vi "Main.vi"(11 "Module Admin":refnum<class "Delacor_lib_QMH_Module Admin.lvclass">) -> ()   [LabVIEW 2025, in "ATM Module.lvlib"]
doc: "ATM machine made with a DQMH module.\n\nTakes user input in the form of a PIN to verify account.\n\nShows balance. Facilitates withdraw, deposit, and \"Fast Cash\" $50 withdrawals."
uses:
  ATM Module.lvlib
  <vilib>/Delacor/Delacor QMH/Libraries/Module Admin_class/Delacor_lib_QMH_Module Admin.lvclass
  Controls/FP Data Refs.ctl
  Module Data--cluster.ctl
  Stop Argument--cluster.ctl
  <vilib>/Delacor/Delacor QMH/Libraries/Message Queue_class/Delacor_lib_QMH_Message Queue.lvclass/Delacor_lib_QMH_Message Queue.ctl
  <vilib>/Delacor/Delacor QMH/Libraries/Module Admin_class/Delacor_lib_QMH_Module Admin.lvclass/Delacor_lib_QMH_Module Admin.ctl
  <vilib>/Utility/miscctls.llb/LVPointTypeDef.ctl
  <vilib>/Delacor/Delacor QMH/Libraries/Message Queue_class/Delacor_lib_QMH_Enqueue Message (Single).vi
  <vilib>/Delacor/Delacor QMH/Libraries/Module Admin_class/Delacor_lib_QMH_Get External Launch.vi
  <vilib>/Delacor/Delacor QMH/Libraries/Message Queue_class/Delacor_lib_QMH_Message Queue.lvclass
panel:
  in  "Enter":bool
  in  "User Input":string
  in  "Right Buttons":T1
  out "Right Menu":T2
  in  "Left Buttons":T1
  out "Left Menu":T2
  in  "Card Simulator":bool
  out "ATM Messages":string
  out "error out":errorcluster
  out "Status":string
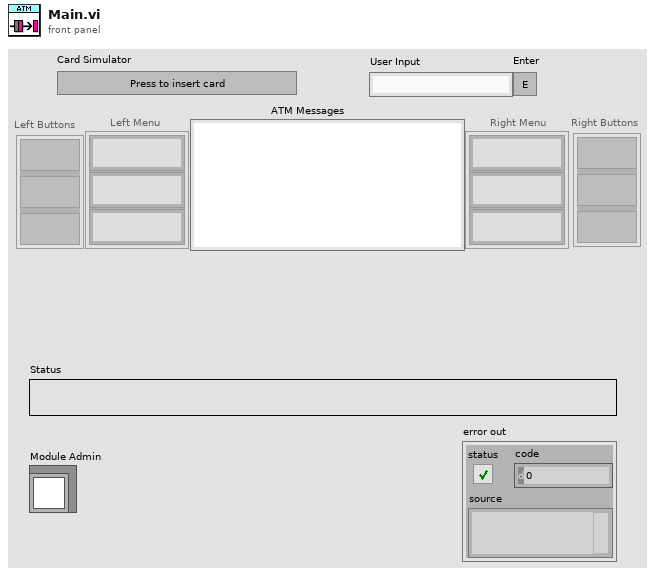
[diagram p1: front panel]
types:
  T1 = cluster{"Func Button":bool, "Func Button 2":bool, "Func Button 3":bool}
  T2 = cluster{"RFS String":string, "RFS String 2":string, "RFS String 3":string}
  T3 = typedef "FP Data Refs.ctl" = cluster{"User Input":refnum<vi>, "Right Buttons":refnum<vi>, "Right Menu":refnum<vi>, "Left Buttons":refnum<vi>, "Left Menu":refnum<vi>, "Enter":refnum<vi>}
  T4 = typedef "ATM Module.lvlib/Request Events--cluster.ctl" = cluster{"Stop Module":refnum<user-event>, "Show Panel":refnum<user-event>, "Hide Panel":refnum<user-event>, "Get Module Execution Status":refnum<user-event>, "Show Diagram":refnum<user-event>, "Private.Reset Timer":refnum<user-event>}
  T5 = typedef "ATM Module.lvlib/Module Data--cluster.ctl" = cluster{"Status":string, "Account PIN":string}
  T6 = enum32{"invalid lock state", "Not Locked", "Locked (No Password)", "Password-protected"}
  T7 = typedef "ATM Module.lvlib/Stop Argument--cluster.ctl" = cluster{"Origin":string, "Exit via Stop Module Req?":bool, "Wait for Module to stop?":bool}
  T8 = typedef "LVPointTypeDef.ctl" = cluster{"Horizontal":i16, "Vertical":i16}
  T9 = enum32{"Invalid", "Standard", "Closed", "Hidden", "Minimized", "Maximized"}
  T10 = enum8{"Enabled", "Disabled", "Disabled and Grayed Out"}
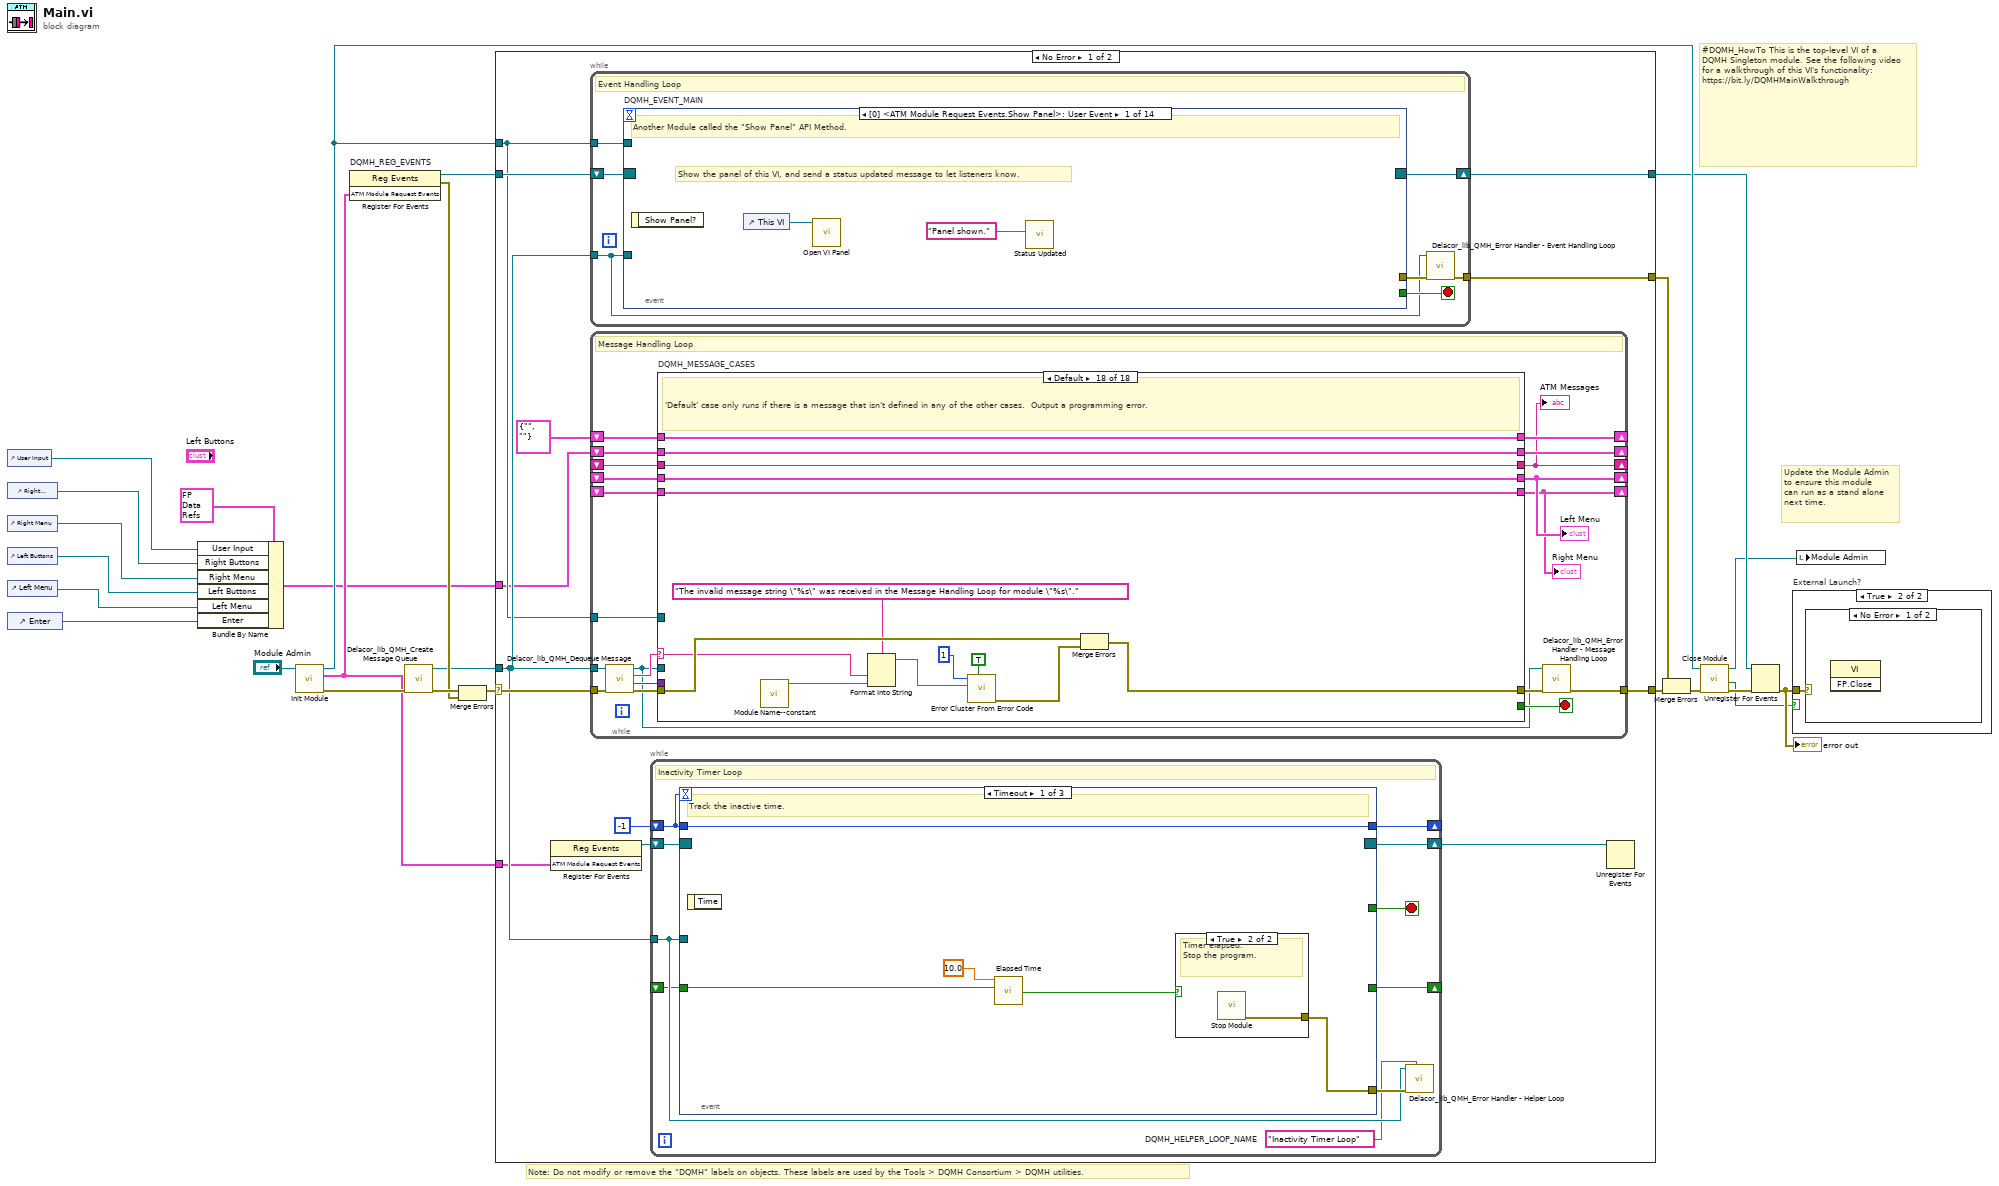
[diagram p0: block diagram]
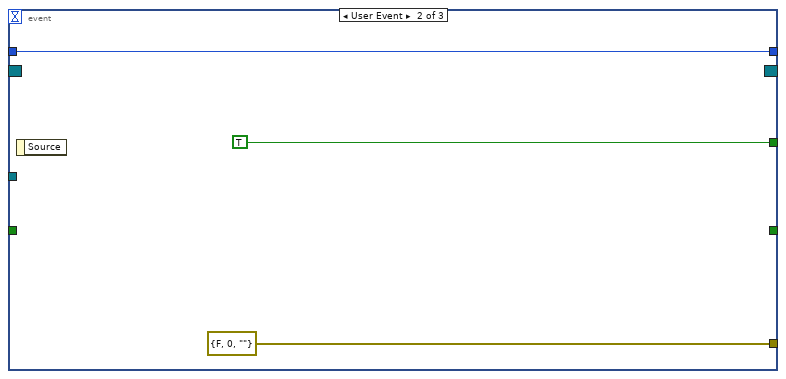
[diagram p3: hidden frame]
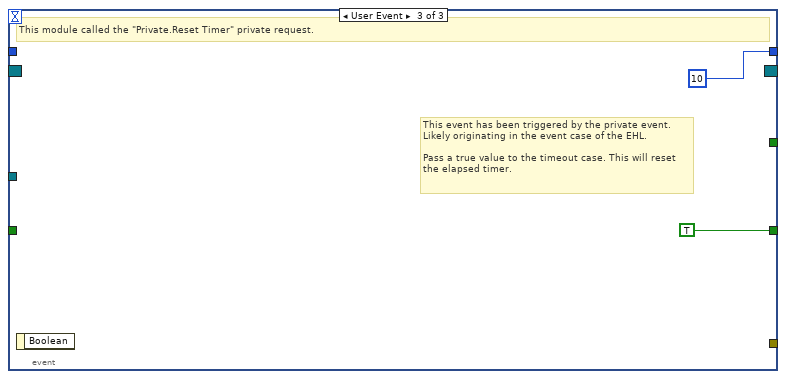
[diagram p4: hidden frame]
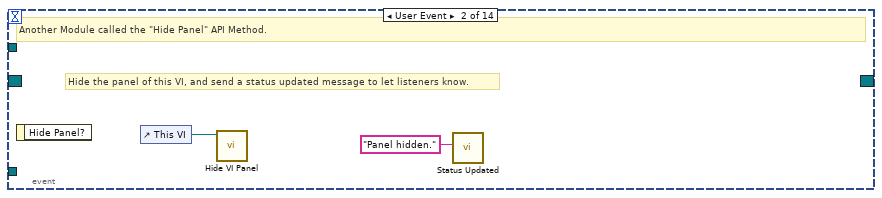
[diagram p5: hidden frame]
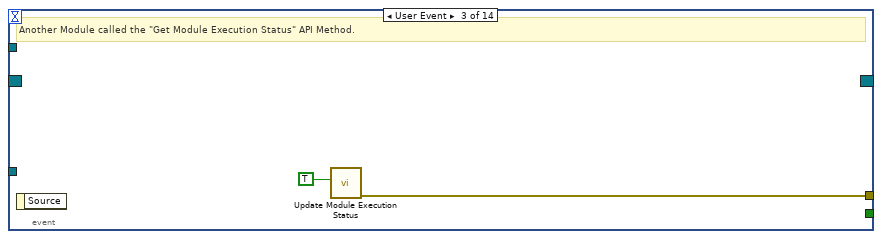
[diagram p6: hidden frame]
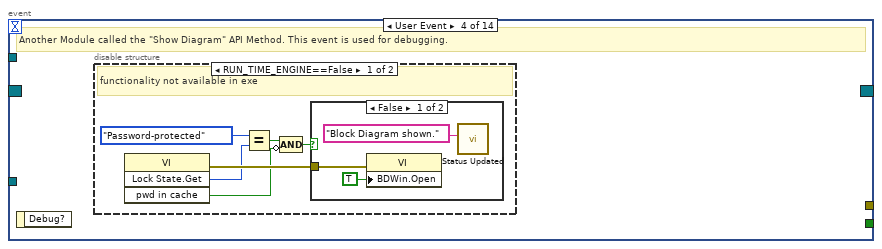
[diagram p7: hidden frame]
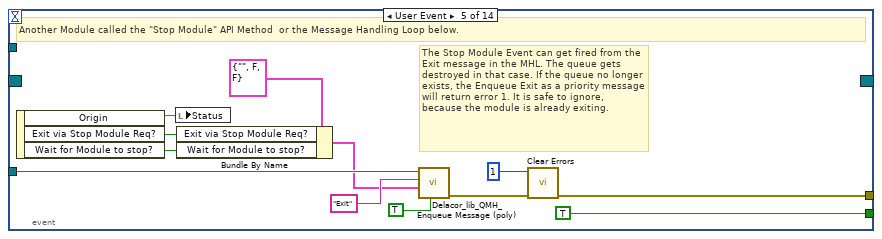
[diagram p10: hidden frame]
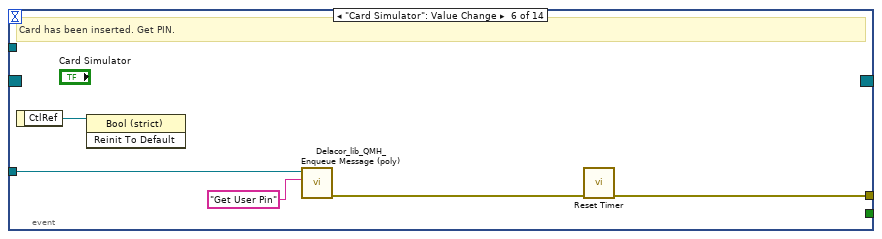
[diagram p11: hidden frame]
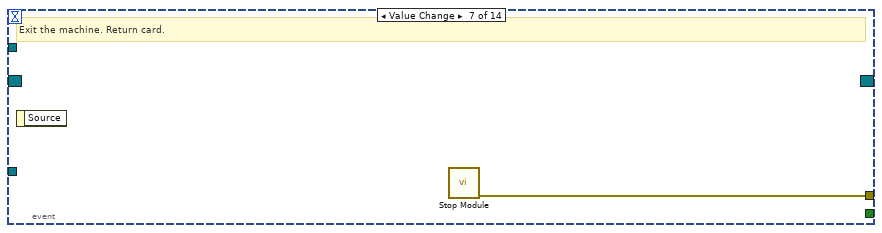
[diagram p12: hidden frame]
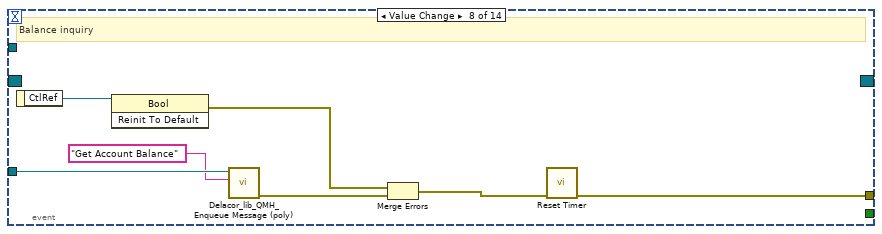
[diagram p13: hidden frame]
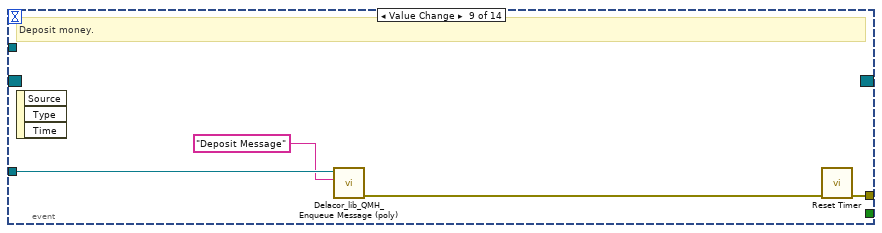
[diagram p14: hidden frame]
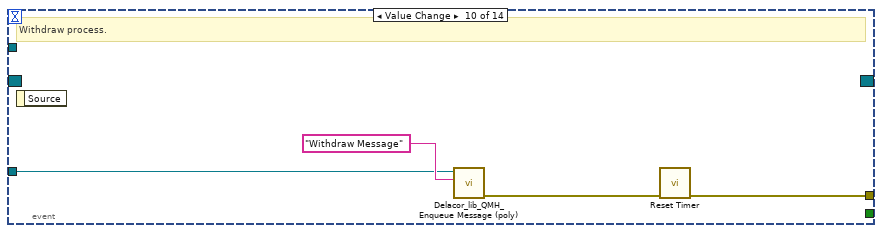
[diagram p15: hidden frame]
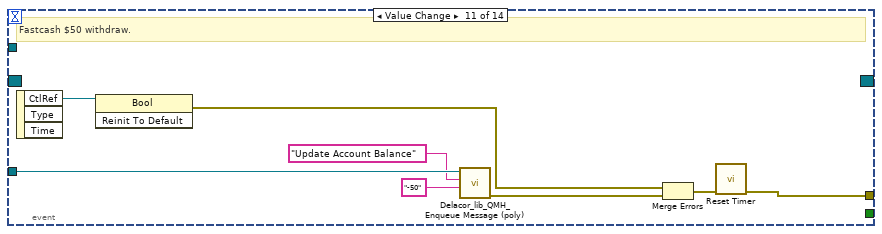
[diagram p16: hidden frame]
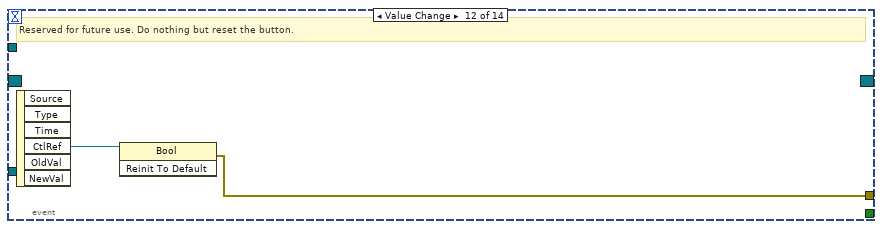
[diagram p17: hidden frame]
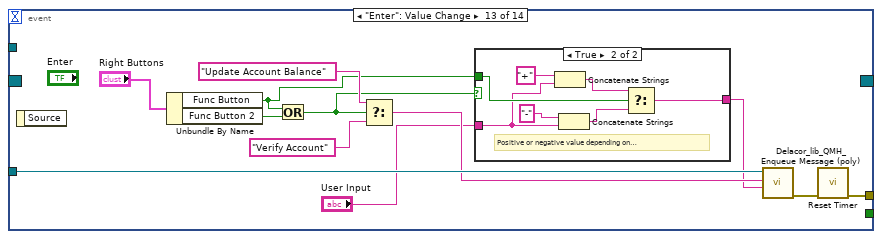
[diagram p18: hidden frame]
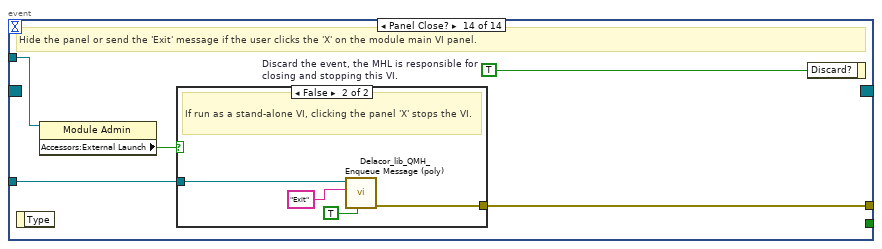
[diagram p20: hidden frame]
diagram:
  # "#DQMH_HowTo This is the top-level VI of a DQMH Singleton module. See the following video for a walkthrough of this VI's functionality: https://bit.ly/DQMHMainWalkthrough"
  # "Note: Do not modify or remove the \"DQMH\" labels on objects. These labels are used by the Tools > DQMH Consortium > DQMH utilities."
  # "Update the Module Admin to ensure this module can run as a stand alone next time."
  n1 = control-ref of="User Input"() -> (w8:refnum<vi>)
  n2 = control-ref of="Right Buttons"() -> (w7:refnum<vi>)
  n3 = control-ref of="Right Menu"() -> (w6:refnum<vi>)
  n4 = control-ref of="Left Buttons"() -> (w5:refnum<vi>)
  n5 = control-ref of="Left Menu"() -> (w4:refnum<vi>)
  n6 = control-ref of="Enter"() -> (w2:refnum<vi>)
  n7 = Bundle By Name(cluster=T3 {"User Input"=refnum, "Right Buttons"=refnum, "Right Menu"=refnum, "Left Buttons"=refnum, "Left Menu"=refnum, "Enter"=refnum}, "User Input"=w8, "Right Buttons"=w7, "Right Menu"=w6, "Left Buttons"=w5, "Left Menu"=w4, "Enter"=w2) -> (w3:T3)
  n8 = call "Init Module.vi"("Singleton Module Admin in"="Module Admin") -> ("error out"=w24:errorcluster, "ATM Module Request Events"=w9:T4, "Singleton Module Admin out"=w16:refnum<class "Delacor_lib_QMH_Module Admin.lvclass">)  [unwired: 8 in]
  n9 = register-events "DQMH_REG_EVENTS"(w9) -> (reference out=w14:refnum<event-registration>, error out=w17:errorcluster)  [unwired: 2 in]
  n10 = call <vilib>:"Delacor_lib_QMH_Create Message Queue.vi"("error in"=w24) -> ("error out"=w19:errorcluster, "Message Queue"=w13:refnum<class "Delacor_lib_QMH_Message Queue.lvclass">)  [unwired: 9 in]
  n11 = Merge Errors(w19, w17) -> (w18:errorcluster)
  n12 = case shown="No Error" w18 {
    selector: w18 -> [w36 w455]
    tunnel: [w38 w454] -> w25
    tunnel: [w35 w453] -> w15
    tunnel: w14 -> [w34 w453]
    tunnel: w13 -> [w33 w448]
    tunnel: [w37 _] -> w22
    tunnel: w16 -> [w32 w449]
    tunnel: w9 -> [w31 _]
    tunnel: w3 -> [w26 _]
    frame No Error {
      n13 = register-events ("DQMH_HELPER_REGFOREVENTS")(w31) -> (reference out=w29:refnum<event-registration>)  [unwired: 2 in, 1 out]
      n14 = while {
        tunnel: w33 -> [w60]
        shift-right: [w63] -> w35
        shift-left: w34 -> [w64]
        tunnel: [w65] -> w37
        tunnel: w32 -> [w61]
        stop <- w62 stop-if-true
        # "Event Handling Loop"
        n15 = event "DQMH_EVENT_MAIN" shown="[0] <ATM Module Request Events.Show Panel>: User Event" {
          selector: w64 -> [_ _ _ _ _ _ _ _ _ _ _ _ _ _]
          dyn-events: [_ _ _ _ _ _ _ _ _ _ _ _ _ _] -> w63
          timeout: _ -> [_ _ _ _ _ _ _ _ _ _ _ _ _ _]
          tunnel: [_ _ _ _ TRUE ("Discard?") _ _ _ _ _ _ _ _ _] -> w62
          tunnel: w60 -> [_ _ _ _ w89 w98 _ w105 w110 w112 w121 _ w132 w147]
          tunnel: [_ _ w72 _ w92 w94 w99 w102 w107 w111 w115 w123 w129 w149] -> w66
          tunnel: w61 -> [_ _ _ _ _ _ _ _ _ _ _ _ _ w146]
          event User Event {
            # "Show the panel of this VI, and send a status updated message to let listeners know."
            # "Another Module called the \"Show Panel\" API Method."
            n16 = event-data() -> ()  [unwired: 1 in, 1 out]
            n17 = control-ref of="This VI"() -> (w68:refnum<vi>)
            n18 = call "Open VI Panel.vi"("VI"=w68) -> ()  [unwired: 10 in, 1 out]
            n19 = call "Status Updated.vi"("Status"="Panel shown." ("format string")) -> ()  [unwired: 10 in, 1 out]
          }
          event User Event {
            # "Hide the panel of this VI, and send a status updated message to let listeners know."
            # "Another Module called the \"Hide Panel\" API Method."
            n20 = event-data() -> ()  [unwired: 1 in, 1 out]
            n21 = control-ref of="This VI"() -> (w70:refnum<vi>)
            n22 = call "Hide VI Panel.vi"("VI"=w70) -> ()  [unwired: 10 in, 1 out]
            n23 = call "Status Updated.vi"("Status"="Panel hidden." ("format string")) -> ()  [unwired: 10 in, 1 out]
          }
          event User Event {
            # "Another Module called the \"Get Module Execution Status\" API Method."
            n24 = event-data() -> ()  [unwired: 1 in, 1 out]
            n25 = call "Update Module Execution Status.vi"("Running?"=TRUE) -> ("error out"=w72:errorcluster)  [unwired: 10 in]
          }
          event User Event {
            # "Another Module called the \"Show Diagram\" API Method. This event is used for debugging."
            n26 = event-data() -> ()  [unwired: 1 in, 1 out]
            n27 = disable-structure shown="RUN_TIME_ENGINE==False" {
              frame condition #0 (active) {
                # "functionality not available in exe"
                n28 = invoke on="Invoke Node" class="VI" method="Lock State.Get"() -> (error out=w78:errorcluster, "Get Lock State"=w77:T6, "pwd in cache"=w74:bool)  [unwired: 4 in, 1 out]
                n29 = Equal?(x=T6."Password-protected", y=w77) -> (x = y?=w75:bool)
                n30 = Compound Arithmetic op=AND(w75, invert w74) -> (w73:bool)
                n31 = case shown="False" w73 {
                  tunnel: w78 -> [w81 _]
                  frame False {
                    n32 = property on="Property Node" class="VI"(error in=w81, "BDWin.Open"=TRUE ("Block Diagram Window:Open")) -> ()  [unwired: 1 in, 2 out]
                    n33 = call "Status Updated.vi"("Status"="Block Diagram shown." ("format string")) -> ()  [unwired: 10 in, 1 out]
                  }
                  frame True {
                    # "Password-protected VI, and the password is not in the cache. Do not show the diagram."
                  }
                }
              }
              frame condition #1 {
              }
            }
          }
          event User Event {
            # "The Stop Module Event can get fired from the Exit message in the MHL. The queue gets destroyed in that case. If the queue no longer exists, the Enqueue Exit as a priority message will return error 1. It is safe to ignore, because the module is already exiting."
            # "Another Module called the \"Stop Module\" API Method  or the Message Handling Loop below."
            n34 = event-data() -> ("Origin"=w88:string, "Exit via Stop Module Req?"=w84:bool, "Wait for Module to stop?"=w83:bool)  [unwired: 1 in]
            n35 = local write "Status"(w88) -> ()
            n36 = Bundle By Name(cluster=T7 {"Origin"="", "Exit via Stop Module Req?"=FALSE, "Wait for Module to stop?"=FALSE} ("Stop Argument"), "Exit via Stop Module Req?"=w84, "Wait for Module to stop?"=w83) -> (w82:T7)
            n37 = call-poly <vilib>:"Delacor_lib_QMH_Enqueue Message (poly).vi"("Priority Message? (F)"=TRUE, "Message Data"=w82, "Message"="Exit", "Message Queue in"=w89) -> ("error out"=w93:errorcluster)  [unwired: 6 in, 1 out]
            n38 = call <vilib>:"Clear Errors.vi"("error in (no error)"=w93, "specific error code to clear (0: all)"=1) -> ("error out"=w92:errorcluster)  [unwired: 4 in, 1 out]
          }
          event "Card Simulator": Value Change {
            # "Card has been inserted. Get PIN."
            n39 = event-data() -> ("CtlRef"=w95:refnum<vi>)  [unwired: 1 in]
            n40 = invoke on="Invoke Node" class="Bool (strict)" method="Reinit To Default"(reference=w95) -> ()  [unwired: 2 in, 3 out]
            n41 = call-poly <vilib>:"Delacor_lib_QMH_Enqueue Message (poly).vi"("Message"="Get User Pin", "Message Queue in"=w98) -> ("error out"=w97:errorcluster)  [unwired: 8 in, 1 out]
            n42 = call "Reset Timer.vi"("error in"=w97) -> ("error out"=w94:errorcluster)  [unwired: 10 in]
          }
          event "Left Buttons.Func Button 3": Value Change {
            # "Exit the machine. Return card."
            n43 = event-data() -> ()  [unwired: 1 in, 1 out]
            n44 = call "Stop Module.vi"() -> ("error out"=w99:errorcluster)  [unwired: 11 in]
          }
          event "Left Buttons.Func Button 2": Value Change {
            # "Balance inquiry"
            n45 = event-data() -> ("CtlRef"=w106:refnum<vi>)  [unwired: 1 in]
            n46 = invoke on="Invoke Node" class="Bool" method="Reinit To Default"(reference=w106) -> (error out=w100:errorcluster)  [unwired: 2 in, 2 out]
            n47 = call-poly <vilib>:"Delacor_lib_QMH_Enqueue Message (poly).vi"("Message"="Get Account Balance", "Message Queue in"=w105) -> ("error out"=w103:errorcluster)  [unwired: 8 in, 1 out]
            n48 = Merge Errors(w100, w103) -> (w101:errorcluster)
            n49 = call "Reset Timer.vi"("error in"=w101) -> ("error out"=w102:errorcluster)  [unwired: 10 in]
          }
          event "Right Buttons.Func Button": Value Change {
            # "Deposit money."
            n50 = event-data() -> ()  [unwired: 1 in, 3 out]
            n51 = call-poly <vilib>:"Delacor_lib_QMH_Enqueue Message (poly).vi"("Message"="Deposit Message", "Message Queue in"=w110) -> ("error out"=w109:errorcluster)  [unwired: 8 in, 1 out]
            n52 = call "Reset Timer.vi"("error in"=w109) -> ("error out"=w107:errorcluster)  [unwired: 10 in]
          }
          event "Right Buttons.Func Button 2": Value Change {
            # "Withdraw process."
            n53 = event-data() -> ()  [unwired: 1 in, 1 out]
            n54 = call-poly <vilib>:"Delacor_lib_QMH_Enqueue Message (poly).vi"("Message"="Withdraw Message", "Message Queue in"=w112) -> ("error out"=w113:errorcluster)  [unwired: 8 in, 1 out]
            n55 = call "Reset Timer.vi"("error in"=w113) -> ("error out"=w111:errorcluster)  [unwired: 10 in]
          }
          event "Right Buttons.Func Button 3": Value Change {
            # "Fastcash $50 withdraw."
            n56 = event-data() -> ("CtlRef"=w118:refnum<vi>)  [unwired: 1 in, 2 out]
            n57 = invoke on="Invoke Node" class="Bool" method="Reinit To Default"(reference=w118) -> (error out=w116:errorcluster)  [unwired: 2 in, 2 out]
            n58 = call-poly <vilib>:"Delacor_lib_QMH_Enqueue Message (poly).vi"("Message Data"="-50", "Message"="Update Account Balance" ("t"), "Message Queue in"=w121) -> ("error out"=w122:errorcluster)  [unwired: 7 in, 1 out]
            n59 = Merge Errors(w116, w122) -> (w117:errorcluster)
            n60 = call "Reset Timer.vi"("error in"=w117) -> ("error out"=w115:errorcluster)  [unwired: 10 in]
          }
          event "Left Buttons.Func Button": Value Change {
            # "Reserved for future use. Do nothing but reset the button."
            n61 = event-data() -> ("CtlRef"=w124:refnum<vi>)  [unwired: 1 in, 5 out]
            n62 = invoke on="Invoke Node" class="Bool" method="Reinit To Default"(reference=w124) -> (error out=w123:errorcluster)  [unwired: 2 in, 2 out]
          }
          event "Enter": Value Change {
            n63 = event-data() -> ()  [unwired: 1 in, 1 out]
            n64 = Unbundle By Name("Right Buttons") -> ("Func Button"=w127:bool, "Func Button 2"=w135:bool)
            n65 = Or(x=w127, y=w135) -> (x .or. y?=w128:bool)
            n66 = Select(t="Update Account Balance", s=w128, f="Verify Account") -> (s? t:f=w131:string)
            n67 = case shown="True" w128 {
              tunnel: w127 -> [_ w139]
              tunnel: "User Input" -> [w137 w138]
              tunnel: [w137 w140] -> w125
              frame False {
              }
              frame True {
                # "Positive or negative value depending on\ndeposit or withdraw."
                n68 = Concatenate Strings("+" ("string"), w138) -> (w141:string)
                n69 = Concatenate Strings("-" ("string"), w138) -> (w142:string)
                n70 = Select(t=w141, s=w139, f=w142) -> (s? t:f=w140:string)
              }
            }
            n71 = call-poly <vilib>:"Delacor_lib_QMH_Enqueue Message (poly).vi"("Message Data"=w125, "Message"=w131, "Message Queue in"=w132) -> ("error out"=w130:errorcluster)  [unwired: 7 in, 1 out]
            n72 = call "Reset Timer.vi"("error in"=w130) -> ("error out"=w129:errorcluster)  [unwired: 10 in]
          }
          event Panel Close? {
            w148 = TRUE  # Discard the event, the MHL is responsible for closing and stopping this VI.
            # "Hide the panel or send the 'Exit' message if the user clicks the 'X' on the module main VI panel."
            n73 = event-data() -> ()  [unwired: 1 in, 1 out]
            n74 = property on="Property Node" class="Module Admin"(reference=w146) -> ("Accessors:External Launch"=w145:bool)  [unwired: 1 in, 2 out]
            n75 = case shown="False" w145 {
              tunnel: w147 -> [_ w155]
              tunnel: [_ w156] -> w149
              frame True {
                # "If externally launched, clicking the 'X' hides the panel, but doesn't close it."
                n76 = control-ref of="This VI"() -> (w152:refnum<vi>)
                n77 = call "Hide VI Panel.vi"("VI"=w152) -> ("error out"=w150:errorcluster)  [unwired: 10 in]
                n78 = call "Status Updated.vi"("error in"=w150, "Status"="Panel hidden." ("format string")) -> ()  [unwired: 9 in, 1 out]
              }
              frame False {
                # "If run as a stand-alone VI, clicking the panel 'X' stops the VI."
                n79 = call-poly <vilib>:"Delacor_lib_QMH_Enqueue Message (poly).vi"("Priority Message? (F)"=TRUE, "Message"="Exit", "Message Queue in"=w155) -> ("error out"=w156:errorcluster)  [unwired: 7 in, 1 out]
              }
            }
            n80 = event-data ("Event Filter Node")("Discard?"=w148) -> ()  [unwired: 1 in, 1 out]
          }
        }
        n81 = call-dynamic "Delacor_lib_QMH_Error Handler - Event Handling Loop.vi"("error in"=w66, "Message Queue in"=w60) -> ("dup error in"=w65:errorcluster)  [unwired: 8 in, 1 out]
      }
      n82 = while {
        tunnel: w33 -> [w165]
        shift-right: [w173] -> _
        shift-left: T5 {"Status"="", "Account PIN"=""} ("Data Cluster") -> [w174]
        tunnel: w36 -> [w176]
        tunnel: [w168] -> w38
        tunnel: w32 -> [w169]
        shift-right: [w163] -> _
        shift-left: w26 -> [w164]
        shift-right: [w162] -> _
        shift-left: _ -> [w161]
        shift-right: [w160] -> _
        shift-left: _ -> [w159]
        shift-right: [w158] -> _
        shift-left: _ -> [w157]
        stop <- w172 stop-if-true
        # "Message Handling Loop"
        n83 = call-dynamic "Delacor_lib_QMH_Dequeue Message.vi"("error in"=w176, "Message Queue in"=w165) -> ("error out"=w175:errorcluster, "Message Data"=w170:variant, "Message"=w171:string, "Message Queue out"=w166:refnum<class "Delacor_lib_QMH_Message Queue.lvclass">)  [unwired: 6 in]
        n84 = case "DQMH_MESSAGE_CASES" shown="Default" w171 {
          selector: w171 -> [_ _ _ _ _ _ _ _ _ _ _ _ _ _ _ _ _ w443]
          tunnel: w166 -> [w186 _ _ _ _ _ _ _ w306 w319 _ _ _ _ _ w401 w427 _]
          tunnel: w175 -> [w205 w213 w220 w228 w236 w255 w287 w298 w311 w328 w351 w362 w374 w380 w393 w408 w433 w446]
          tunnel: [w204 w213 w219 w224 w230 w240 w286 w298 w303 w323 w351 w362 w371 w380 w392 w404 w428 w447] -> w167
          tunnel: w174 -> [w195 w212 w218 w227 w235 w254 w289 w297 w310 w314 w350 w361 w373 w379 w390 w403 w426 w444]
          tunnel: [w194 w212 w218 w227 w235 w254 w289 w297 w310 w313 w350 w361 w373 w379 w390 w403 w426 w444] -> w173
          tunnel: [_ _ _ _ _ _ _ _ _ _ _ _ _ _ _ _ w425 _] -> w172
          tunnel: w170 -> [_ _ _ _ _ w252 _ _ _ w326 _ _ w368 _ _ w402 w424 _]
          tunnel: w169 -> [w196 _ _ _ _ _ _ _ _ _ _ _ _ _ _ w400 w419 _]
          tunnel: w164 -> [w185 w211 w217 w222 w231 w250 w292 w296 w309 w327 w349 w360 w372 w378 w384 w397 w418 w437]
          tunnel: [w185 w211 w217 w222 w231 w250 w292 w296 w309 w327 w349 w360 w372 w378 w384 w397 w418 w437] -> w163
          tunnel: ["Welcome to Acme Bank.\nPlease insert your card\nand enter your account\nnumber in the User Input.\n\nPress Enter (E) when done." w210 w216 "Please enter amount to withdraw and press\nEnter (E) when done" "Please enter amount to deposit and press\nEnter (E) when done" w238 w283 w295 w308 w322 w348 w356 w365 w377 w383 w396 "Your session has been terminated\ndue to inactivity or menu selection.\nPlease take your card\n\nGoodbye!" w436] -> w162
          tunnel: w161 -> [_ w210 w216 _ _ _ _ w295 w308 _ w348 w356 w365 w377 w383 w396 _ w436]
          tunnel: [w182 w209 w215 w226 w234 w257 w291 T2 {"RFS String"="", "RFS String 2"="", "RFS String 3"=""} ("Left Menu") w300 w316 T2 {"RFS String"="None", "RFS String 2"="Balance Inquiry", "RFS String 3"="Return card\n& Terminate"} ("Left Menu") w353 w364 w376 w382 w395 w417 w435] -> w160
          tunnel: w159 -> [w182 w209 w215 w226 w234 w257 w291 _ w300 w316 _ w353 w364 w376 w382 w395 w417 w435]
          tunnel: [w181 w208 w214 w225 w233 w256 w290 T2 {"RFS String"="", "RFS String 2"="", "RFS String 3"=""} ("Right Menu") w299 w315 T2 {"RFS String"="Deposit", "RFS String 2"="Withdraw", "RFS String 3"="Fast Cash $50"} ("Right Menu") w352 w363 w375 w381 w394 w416 w434] -> w158
          tunnel: w157 -> [w181 w208 w214 w225 w233 w256 w290 _ w299 w315 _ w352 w363 w375 w381 w394 w416 w434]
          frame "Initialize" {
            w190 = "Initial Message" ("Initial Message")
            # "#DQMH_CodeNeeded - Initialize the appearance of the front panel."
            # "#DQMH_CodeNeeded - Initialize your state data here."
            # "Initialize - Any operation that needs to be done before the module can receive messages. Synchronize Caller Events.vi will inform Start Module.vi that the module has launched and is ready to receive messages. Module Did Init.vi will broadcast that the module initialized."
            n85 = call "Synchronize Caller Events.vi"("error in"=w205, "Singleton Module Admin in"=w196) -> ("error out"=w188:errorcluster, "Singleton Module Admin out"=w191:refnum<class "Delacor_lib_QMH_Module Admin.lvclass">)  [unwired: 8 in]
            n86 = property on="Property Node" class="Module Admin"(reference=w191) -> ("Accessors:External Launch"=w200:bool)  [unwired: 1 in, 2 out]
            n87 = Select(t=T9."Hidden" ("State"), s=w200, f=T9."Standard" ("State")) -> (s? t:f=w197:T9)
            n88 = call "Module Name--constant.vi"() -> ("Module Name"=w203:string)  [unwired: 11 in]
            n89 = property on="Property Node" class="VI"("Front Panel.Title"=w203) -> (reference out=w202:refnum<vi>, error out=w207:errorcluster)  [unwired: 2 in]
            n90 = invoke on="Invoke Node" class="VI" method="FP.Open"(reference=w202, error in=w207, "State"=w197) -> (reference out=w201:refnum<vi>, error out=w206:errorcluster)  [unwired: 2 in, 3 out]
            n91 = Bundle By Name(cluster=w195, "Status"=w190) -> (w194:T5)
            n92 = call-poly <vilib>:"Delacor_lib_QMH_Enqueue Message (poly).vi"("error in"=w188, "Message"="Reset to Defaults", "Message Queue in"=w186) -> ("error out"=w180:errorcluster, "Message Queue out"=w178:refnum<class "Delacor_lib_QMH_Message Queue.lvclass">)  [unwired: 7 in]
            n93 = invoke on="Invoke Node" class="VI" method="FP.Center"(reference=w201, error in=w206) -> ()  [unwired: 1 in, 3 out]
            n94 = property on="Pane" class="Pane"("Origin"=T8 {"Horizontal"=0, "Vertical"=0}) -> ()  [unwired: 2 in, 2 out]
            n95 = call-poly <vilib>:"Delacor_lib_QMH_Enqueue Message (poly).vi"("error in"=w180, "Message"="Depopulate Menus", "Message Queue in"=w178) -> ("error out"=w179:errorcluster)  [unwired: 7 in, 1 out]
            n96 = call "Reset Timer.vi"("error in"=w179) -> ("error out"=w187:errorcluster)  [unwired: 10 in]
            n97 = call "Module Name--constant.vi"() -> ("Module Name"=w192:string)  [unwired: 11 in]
            n98 = call "Module Did Init.vi"("error in"=w187, "Initialized?"=TRUE, "Origin"=w192) -> ("error out"=w204:errorcluster)  [unwired: 8 in]
            "Status" <- w190
          }
          frame "---Module Specific---" {
            # "Separator -- The following cases handle messages specific to this Module."
          }
          frame "---Copy This Frame---" {
            # "Duplicate this frame when creating new messages.  Change this comment in the duplicated frame to describe this message."
            n99 = Merge Errors(w220) -> (w219:errorcluster)
          }
          frame "Withdraw Message" {
            n100 = call "Prepare User Input.vi"("cluster"=w222) -> ("error out"=w223:errorcluster)  [unwired: 10 in]
            n101 = Merge Errors(w223, w228) -> (w224:errorcluster)
          }
          frame "Deposit Message" {
            n102 = call "Prepare User Input.vi"("cluster"=w231) -> ("error out"=w229:errorcluster)  [unwired: 10 in]
            n103 = Merge Errors(w229, w236) -> (w230:errorcluster)
          }
          frame "Update Account Balance" {
            n104 = Variant To Data(error in=w255, type="" ("Empty String Constant"), Variant=w252) -> (data=w249:string, error out=w253:errorcluster)
            n105 = Unbundle By Name(w254) -> ("Account PIN"=w241:string)
            n106 = Fract/Exp String To Number(string=w249) -> (number=w247:dbl)  [unwired: 3 in, 1 out]
            n107 = Greater Than 0?(x=w247) -> (x > 0?=w248:bool)
            n108 = call "Get Account Info.vi"("error in"=w253, "PIN"=w241) -> ("error out"=w242:errorcluster, "Account Balance"=w246:string)  [unwired: 6 in, 2 out]
            n109 = Fract/Exp String To Number(string=w246) -> (number=w245:dbl)  [unwired: 3 in, 1 out]
            n110 = case shown="False" w248 {
              selector: w248 -> [w275 w280]
              tunnel: w247 -> [w273 w278]
              tunnel: w245 -> [w277 w282]
              tunnel: [w276 TRUE] -> w244
              tunnel: [w273 w278] -> w243
              tunnel: [w275 w280] -> w239
              tunnel: [w274 w279] -> w237
              frame False {
                # "Money left in the account?"
                # "Negative number. This is a withdraw."
                n111 = Add(x=w277, y=w273) -> (x+y=w274:dbl)
                n112 = Greater Than 0?(x=w274) -> (x > 0?=w276:bool)
              }
              frame True {
                # "Positive Number. This is a deposit."
                n113 = Add(x=w278, y=w282) -> (x+y=w279:dbl)
              }
            }
            n114 = case shown="True" w244 {
              tunnel: w243 -> [_ w268]
              tunnel: w242 -> [w259 w272]
              tunnel: w241 -> [_ w271]
              tunnel: [w259 w270] -> w240
              tunnel: w239 -> [_ w269]
              tunnel: ["Insufficient funds in account\nPlease check your balance\nand try again" w262] -> w238
              tunnel: w237 -> [_ w261]
              frame False {
              }
              frame True {
                n115 = Number To Fractional String(number=w268, precision (6)=i16 2) -> (F-format string=w264:string)  [unwired: 2 in]
                n116 = call "Update Account Balance.vi"("error in (no error)"=w272, "Account PIN"=w271, "New Amount"=w261) -> ("error out"=w270:errorcluster)  [unwired: 8 in]
                n117 = Format Into String(format string="$%s Deposited", w264) -> (resulting string=w266:string)  [unwired: 2 in, 1 out]
                n118 = Format Into String(format string="$%s Withdrawn", w264) -> (resulting string=w263:string)  [unwired: 2 in, 1 out]
                n119 = Select(t=w266, s=w269, f=w263) -> (s? t:f=w262:string)
              }
            }
          }
          frame "Get Account Balance" {
            n120 = Unbundle By Name(w289) -> ("Account PIN"=w288:string)
            n121 = call "Get Account Info.vi"("error in"=w287, "PIN"=w288) -> ("error out"=w286:errorcluster, "Account Balance"=w284:string)  [unwired: 6 in, 2 out]
            n122 = Format Into String(format string="Your Balance Is:\n$%s", w284) -> (resulting string=w283:string)  [unwired: 2 in, 1 out]
          }
          frame "Depopulate Menus" {
          }
          frame "Reset to Defaults" {
            n123 = call-poly <vilib>:"Delacor_lib_QMH_Enqueue Message (poly).vi"("error in"=w311, "Message Data"=T10."Disabled and Grayed Out" ("Disabled"), "Message"="Disable Enable All Controls", "Message Queue in"=w306) -> ("error out"=w307:errorcluster)  [unwired: 6 in, 1 out]
            n124 = control-ref of="This VI"() -> (w304:refnum<vi>)
            n125 = invoke on="Invoke Node" class="VI" method="Default Vals.Reinit All"(reference=w304) -> (error out=w302:errorcluster)  [unwired: 2 in, 2 out]
            n126 = Merge Errors(w302, w307) -> (w303:errorcluster)
          }
          frame "Verify Account" {
            n127 = Variant To Data(error in=w328, type="" ("Empty String Constant"), Variant=w326) -> (data=w312:string, error out=w324:errorcluster)
            n128 = call "Get Account Info.vi"("PIN"=w312) -> ("error out"=w317:errorcluster, "Verified?"=w321:bool, "Account Name"=w320:string)  [unwired: 7 in, 1 out]
            n129 = case shown="True" w321 {
              tunnel: ["Account Information Incorrect\nPlease Re-Enter Account Number.\nPress Enter (E) when done" w344] -> w322
              tunnel: w320 -> [_ w343]
              tunnel: w319 -> [_ w342]
              tunnel: [w330 w337] -> w318
              tunnel: w317 -> [w330 w341]
              tunnel: w314 -> [w329 w334]
              tunnel: [w329 w333] -> w313
              tunnel: w312 -> [_ w332]
              frame False {
              }
              frame True {
                n130 = Format Into String(format string="Welcome to Acme Bank\n%s\n\nPlease select transaction\nby using the buttons.", w343) -> (resulting string=w344:string)  [unwired: 2 in, 1 out]
                n131 = call-poly <vilib>:"Delacor_lib_QMH_Enqueue Message (poly).vi"("error in"=w341, "Message Data"=T10."Enabled" ("Disabled"), "Message"="Disable Enable All Controls", "Message Queue in"=w342) -> ("error out"=w338:errorcluster, "Message Queue out"=w335:refnum<class "Delacor_lib_QMH_Message Queue.lvclass">)  [unwired: 6 in]
                n132 = Bundle By Name(cluster=w334, "Account PIN"=w332) -> (w333:T5)
                n133 = call-poly <vilib>:"Delacor_lib_QMH_Enqueue Message (poly).vi"("error in"=w338, "Message"="Populate Menus", "Message Queue in"=w335) -> ("error out"=w337:errorcluster)  [unwired: 7 in, 1 out]
              }
            }
            n134 = Merge Errors(w318, w324) -> (w323:errorcluster)
          }
          frame "Populate Menus" {
          }
          frame "Get User Pin" {
            w354 = T10."Enabled" ("Disabled")
            n135 = Unbundle By Name(w360) -> ("Enter"=w355:refnum<vi>, "User Input"=w359:refnum<vi>)
            n136 = property on="Property Node" class="Bool"(reference=w355, "DisabledEnum"=w354) -> ()  [unwired: 1 in, 2 out]
            n137 = property on="Property Node" class="Str"(reference=w359, "Value"="" ("Empty String Constant"), "DisabledEnum"=w354, "Key Focus"=TRUE) -> ()  [unwired: 1 in, 2 out]
          }
          frame "Disable Enable All Controls" {
            n138 = Variant To Data(error in=w374, type=T10."Enabled" ("Disabled"), Variant=w368) -> (data=w366:T10, error out=w369:errorcluster)
            n139 = call "Enable Disable FP.vi"("Disabled"=w366, "cluster"=w372) -> ("error out"=w370:errorcluster)  [unwired: 9 in]
            n140 = Merge Errors(w370, w369) -> (w371:errorcluster)
          }
          frame "---Exit and Error Handling---" {
            # "Separator - The following cases handle errors and exit messages."
          }
          frame "Simulate MHL Error" {
            # "#DQMH_HowTo The 'Simulate MHL Error' button  illustrates how the MHL handles errors. This event is instructional in nature and can be removed."
            # "Simulate an error occurring at the MHL"
            n141 = call "Module Name--constant.vi"() -> ("Module Name"=w386:string)  [unwired: 11 in]
            n142 = Format Into String(format string="Simulated error originating at Message Handling Loop in %s", w386) -> (resulting string=w387:string)  [unwired: 2 in, 1 out]
            n143 = call <vilib>:"Error Cluster From Error Code.vi"("show call chain? (False)"=TRUE, "error message (\"\")"=w387, "error code (0)"=5001) -> ("error out"=w391:errorcluster)  [unwired: 6 in]
            n144 = Merge Errors(w393, w391) -> (w392:errorcluster)
          }
          frame "Error" {
            # "Error - Check the error message data and respond accordingly. This message is sent by the \"Error Handler\" VIs at the end of each loop in this application."
            n145 = property on="Property Node" class="Module Admin"(reference=w400) -> ("Accessors:External Launch"=w399:bool)  [unwired: 1 in, 2 out]
            n146 = Variant To Data(error in=w408, type=errorcluster {"status"=FALSE, "code"=0, "source"=""} ("error constant"), Variant=w402) -> (data=w398:errorcluster, error out=w406:errorcluster)
            n147 = local write "error out"(w398) -> ()
            n148 = call "Error Reported.vi"("Error"=w398) -> ()  [unwired: 10 in, 1 out]
            n149 = case shown="False" w399 {
              tunnel: [w413 _] -> w405
              tunnel: w401 -> [w411 _]
              tunnel: w398 -> [w412 _]
              frame False {
                n150 = disable-structure "Conditional Disable Structure" shown="Default" {
                  disable-tunnel: w412 -> [w414 _]
                  frame condition #0 (active) {
                    # "If the module is running standalone, then pop up an error dialog and call the \"Exit\" message."
                    n151 = call <vilib>:"Simple Error Handler.vi"("error in (no error)"=w414) -> ()  [unwired: 4 in, 5 out]
                  }
                  frame condition #1 {
                    # "To prevent the Simple Error Handler VI from being loaded (e.g. when deploying to a Real-Time target), add the Conditional Disable Symbol \"DQMH_Disable_SEH\" to your project and set it to TRUE."
                  }
                }
                n152 = call-poly <vilib>:"Delacor_lib_QMH_Enqueue Message (poly).vi"("Priority Message? (F)"=TRUE, "Message"="Exit", "Message Queue in"=w411) -> ("error out"=w413:errorcluster)  [unwired: 7 in, 1 out]
              }
              frame True {
                # "If the module was launched externally, calling the Error Reported broadcast VI is the only action performed by the \"Error\" message. The module's caller can then process the error appropriately."
              }
            }
            n153 = Merge Errors(w406, w405) -> (w404:errorcluster)
          }
          frame "Exit" {
            w423 = 91  # 91: not all Exit messages will have an argument
            w425 = TRUE  # Stop the VI
            # "Release the message queue reference"
            # "Exit - Exit the application."
            n154 = Variant To Data(error in=w433, type=T7 {"Origin"="", "Exit via Stop Module Req?"=FALSE, "Wait for Module to stop?"=FALSE} ("Stop Argument"), Variant=w424) -> (data=w421:T7, error out=w430:errorcluster)
            n155 = call <vilib>:"Clear Errors.vi"("error in (no error)"=w430, "specific error code to clear (0: all)"=w423) -> ("error out"=w432:errorcluster)  [unwired: 4 in, 1 out]
            n156 = control-ref of="This VI"() -> (w420:refnum<vi>)
            n157 = call-dynamic "Delacor_lib_QMH_Release Message Queue.vi"("error in"=w432, "Message Queue"=w427) -> ("error out"=w431:errorcluster)  [unwired: 9 in]
            n158 = call "Handle Exit.vi"("Stop Argument"=w421, "Admin in"=w419, "VI reference"=w420) -> ("error out"=w429:errorcluster)  [unwired: 7 in, 1 out]
            n159 = Merge Errors(w431, w429) -> (w428:errorcluster)
            n160 = call "Error Reported.vi"("Error"=w428) -> ()  [unwired: 10 in, 1 out]
          }
          frame Default {
            # "'Default' case only runs if there is a message that isn't defined in any of the other cases.  Output a programming error."
            n161 = call "Module Name--constant.vi"() -> ("Module Name"=w442:string)  [unwired: 11 in]
            n162 = Format Into String(format string="The invalid message string \"%s\" was received in the Message Handling Loop for module \"%s\".", w443, w442) -> (resulting string=w438:string)  [unwired: 2 in, 1 out]
            n163 = call <vilib>:"Error Cluster From Error Code.vi"("show call chain? (False)"=TRUE, "error message (\"\")"=w438, "error code (0)"=1) -> ("error out"=w445:errorcluster)  [unwired: 6 in]
            n164 = Merge Errors(w446, w445) -> (w447:errorcluster)
          }
        }
        "ATM Messages" <- w162
        "Left Menu" <- w160
        "Right Menu" <- w158
        n165 = call-dynamic "Delacor_lib_QMH_Error Handler - Message Handling Loop.vi"("error in"=w167, "Message Queue in"=w166) -> ("dup error in"=w168:errorcluster)  [unwired: 8 in, 1 out]
      }
      n166 = while "DQMH_HELPER_LOOP" {
        shift-right: [w48] -> _
        shift-left: -1 -> [w47]
        shift-right: [w45] -> w30
        shift-left: w29 -> [w46]
        tunnel: w33 -> [w42]
        shift-right: [w40] -> _
        shift-left: _ -> [w39]
        stop <- w44 stop-if-true
        w41 = "Inactivity Timer Loop"  # DQMH_HELPER_LOOP_NAME
        # "Inactivity Timer Loop"
        n167 = event "DQMH_HELPER_EVENT_STRUCTURE" shown="[0] Timeout" {
          selector: w46 -> [_ _ _]
          dyn-events: [_ _ _] -> w45
          timeout: w47 -> [_ _ _]
          tunnel: w47 -> [w51 w57 _]
          tunnel: [w51 w57 10] -> w48
          tunnel: [_ TRUE _] -> w44
          tunnel: [w49 errorcluster {"status"=FALSE, "code"=0, "source"=""} ("error constant") _] -> w43
          tunnel: w42 -> [_ _ _]
          tunnel: [_ _ TRUE] -> w40
          tunnel: w39 -> [w53 _ _]
          event Timeout {
            # "Track the inactive time."
            n168 = event-data() -> ()  [unwired: 1 in, 1 out]
            n169 = call "Elapsed Time"("Time Target (s)"=10.0, "Reset"=w53) -> ("Time has Elapsed"=w50:bool)  [unwired: 10 in, 7 out]
            n170 = case shown="True" w50 {
              tunnel: [_ w54] -> w49
              frame False {
                # "Not elapsed. Do nothing."
              }
              frame True {
                # "Timer elapsed.\nStop the program."
                n171 = call "Stop Module.vi"() -> ("error out"=w54:errorcluster)  [unwired: 11 in]
              }
            }
          }
          event User Event {
            n172 = event-data() -> ()  [unwired: 1 in, 1 out]
          }
          event User Event {
            # "This event has been triggered by the private event.\nLikely originating in the event case of the EHL.\n\nPass a true value to the timeout case. This will reset\nthe elapsed timer."
            # "This module called the \"Private.Reset Timer\" private request."
            n173 = event-data() -> ()  [unwired: 1 in, 1 out]
          }
        }
        n174 = call-dynamic "Delacor_lib_QMH_Error Handler - Helper Loop.vi"("Error Debug"=w41, "error in"=w43, "Message Queue in"=w42) -> ()  [unwired: 7 in, 2 out]
      }
      n175 = Unregister For Events(event registration refnum=w30) -> ()  [unwired: 1 in, 1 out]
    }
    frame Error {
      # "Synchronize Caller Events.vi will inform Start Module.vi that the module has launched and will let the code calling Start Module.vi register for broadcasts and would permit the caller receive the broadcast that an error occurred at launch time."
      n176 = call-dynamic "Delacor_lib_QMH_Release Message Queue.vi"("error in"=w455, "Message Queue"=w448) -> ("error out"=w454:errorcluster)  [unwired: 9 in]
      n177 = call "Synchronize Caller Events.vi"("Singleton Module Admin in"=w449) -> ("error out"=w456:errorcluster)  [unwired: 9 in, 1 out]
      n178 = call "Module Name--constant.vi"() -> ("Module Name"=w452:string)  [unwired: 11 in]
      n179 = Format Into String(format string="An error occurred during initialization. %s is no longer running.", w452) -> (resulting string=w450:string)  [unwired: 2 in, 1 out]
      n180 = Merge Errors(w454, w456) -> (w457:errorcluster)
      n181 = call "Error Reported.vi"("Additional Information"=w450, "Error"=w457) -> ()  [unwired: 9 in, 1 out]
    }
  }
  n182 = Merge Errors(w22, w25) -> (w21:errorcluster)
  n183 = call "Close Module.vi"("error in"=w21, "Module Admin in"=w16) -> ("error out"=w23:errorcluster, "External Launch"=w10:bool, "Module Admin out"=w11:refnum<class "Delacor_lib_QMH_Module Admin.lvclass">)  [unwired: 7 in]
  n184 = Unregister For Events(event registration refnum=w15, error in=w23) -> (error out=w20:errorcluster)
  "error out" <- w20
  n185 = case "External Launch?" shown="True" w10 {
    tunnel: w20 -> [_ w458]
    frame False {
    }
    frame True {
      n186 = case shown="No Error" w458 {
        frame No Error {
          n187 = invoke on="Invoke Node" class="VI" method="FP.Close"() -> ()  [unwired: 3 in, 3 out]
        }
        frame Error {
          n188 = disable-structure shown="Default" {
            frame condition #0 (active) {
              n189 = invoke on="Invoke Node" class="VI" method="FP.Open"("Activate"=TRUE ("Activate?")) -> ()  [unwired: 4 in, 5 out]
            }
            frame condition #1 {
              # "Don't show panel on error if running inside a built EXE."
            }
          }
        }
      }
    }
  }
  n190 = local write "Module Admin"(w11) -> ()
